vi "Sort sample info metadata.vi"(0 "reference in":refnum<class "metadata.lvclass">, 5 "error in (no error)":errorcluster) -> (14 "reference out":refnum<class "metadata.lvclass">, 16 "Sample info":T1, 19 "error out":errorcluster)   [LabVIEW 2019, in "metadata.lvclass"]
uses:
  metadata.lvclass
  Sample info parameters.ctl
panel:
  out "Array":string[](array[string])
  out "Array 2":i32[](array[numeric])
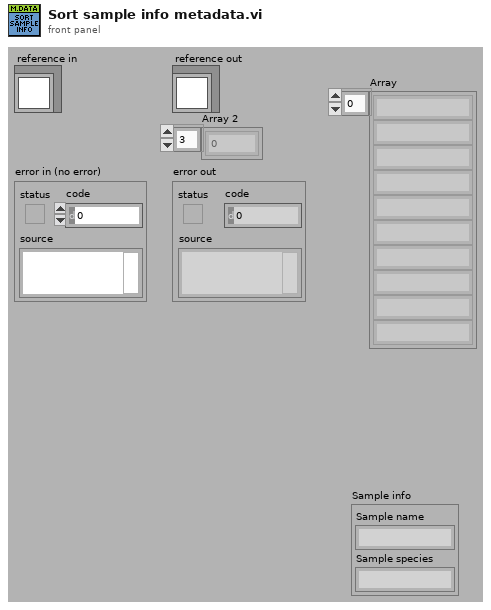
[diagram p1: front panel]
types:
  T1 = typedef "metadata.lvclass/Sample info parameters.ctl" = cluster{"Sample name":string, "Sample species":string}
  T2 = typedef "metadata.lvclass/ObjectAttributesRef.ctl" = refnum<data-value>
  T3 = typedef "metadata.lvclass/ObjectAttributes.ctl" = cluster{"MyAttribute":dbl, "System Control":T4, "file info":T5, "Sample info":T1, "Cantilever info":T6, "XYZ piezos":T7, "Mapping":T8, "Fcurve segment":T9[], "Fast fpga segment":T11, "Chirp":T12, "precision (6)":i16, "width (-)":i16, "Metadata":T13, "config filepath":path, "Section names []":string[], "Property names []":string[], "nb elements":u16}
  T4 = typedef "metadata.lvclass/System control parameters.ctl" = cluster{"FPGA SW version":string, "TDMS file version":string, "Instrument":string, "Instrument model":string, "Instrument scanner":string, "Instrument clockrate (Mhz)":string, "Instrument tick time (us)":string}
  T5 = typedef "metadata.lvclass/File info parameters.ctl" = cluster{"Time Stamp":timestamp, "Filename":string, "Filepath":path, "User":string, "Experiment_name":string, "Curve_id":string, "number_segments":u8, "number_consecutive_scans":u32}
  T6 = typedef "metadata.lvclass/Cantilever info parameters.ctl" = cluster{"spring constant calib method":string, "invOLS calib method":string, "thermal calib deflection channel":string, "model":string, "shape":string, "tip geometry":string, "Laser sum (V)":dbl, "Laser power (mA)":dbl, "invOLS_(nm/V)":dbl, "spring constant nominal (N/m)":dbl, "spring constant calib (N/m)":dbl, "resosnance frequency air calib (Hz)":dbl, "resosnance frequency calib (Hz)":dbl, "quality factor":dbl, "Acoefficident_GCI_(nN.s^1.3/m)":dbl, "half angle (deg)":dbl, "tip radius (m)":dbl, "tip height (m)":dbl, "system mount angle (deg)":dbl}
  T7 = typedef "metadata.lvclass/XYZ piezos parameters.ctl" = cluster{"X stage piezo sensitivity (nm/V)":dbl, "X stage piezo gain":dbl, "X velocity (V/tick)":dbl, "X closed loop":bool, "Y stage piezo sensitivity (nm/V)":dbl, "Y stage piezo gain":dbl, "Y velocity (V/tick)":dbl, "Y closed loop":bool, "Z stage piezo sensitivity (nm/V)":dbl, "Z stage piezo gain":dbl, "Z closed loop":bool, "X position (V)":dbl, "Y position (V)":dbl}
  T8 = typedef "metadata.lvclass/Mapping parameters.ctl" = cluster{"Mapping":bool, "index":u16, "position row":u16, "position column":u16, "next position row":i16, "next position column":i16, "X initial position (V)":dbl, "Y initial position (V)":dbl, "X step size (V)":dbl, "Y step size (V)":dbl}
  T9 = typedef "metadata.lvclass/Fcurve segment.ctl" = cluster{"type":T10, "fast_fpga_trigger":bool, "nb":u8, "duration (ticks)":i64, "nb points":i32, "sampling rate (S/s)":u32, "Zpiezo control out":string, "initial deflection (V)":dbl, "relative setpoint":bool, "setpoint on":bool, "setpoint (V)":dbl, "setpoint trigger channel":string, "velocity (V/tick)":dbl, "Z position setpoint trigger (V)":dbl, "Z retract length (V)":dbl, "dec factor":u32}
  T10 = typedef "metadata.lvclass/Segment type--combobox.ctl" = string
  T11 = typedef "metadata.lvclass/fast fpga segment parameters.ctl" = cluster{"Fast start time trigger":timestamp, "nb_points":u32, "sampling_rate_(S/s)":u32, "duration_(ticks)":u32}
  T12 = typedef "metadata.lvclass/Chirp added parameters.ctl" = cluster{"f start (Hz)":dbl, "f end (Hz)":dbl, "Sweep type":string}
  T13 = typedef "metadata.lvclass/Metadata output --cluster.ctl" = cluster{"Property Names":string[], "Property Values":variant[]}
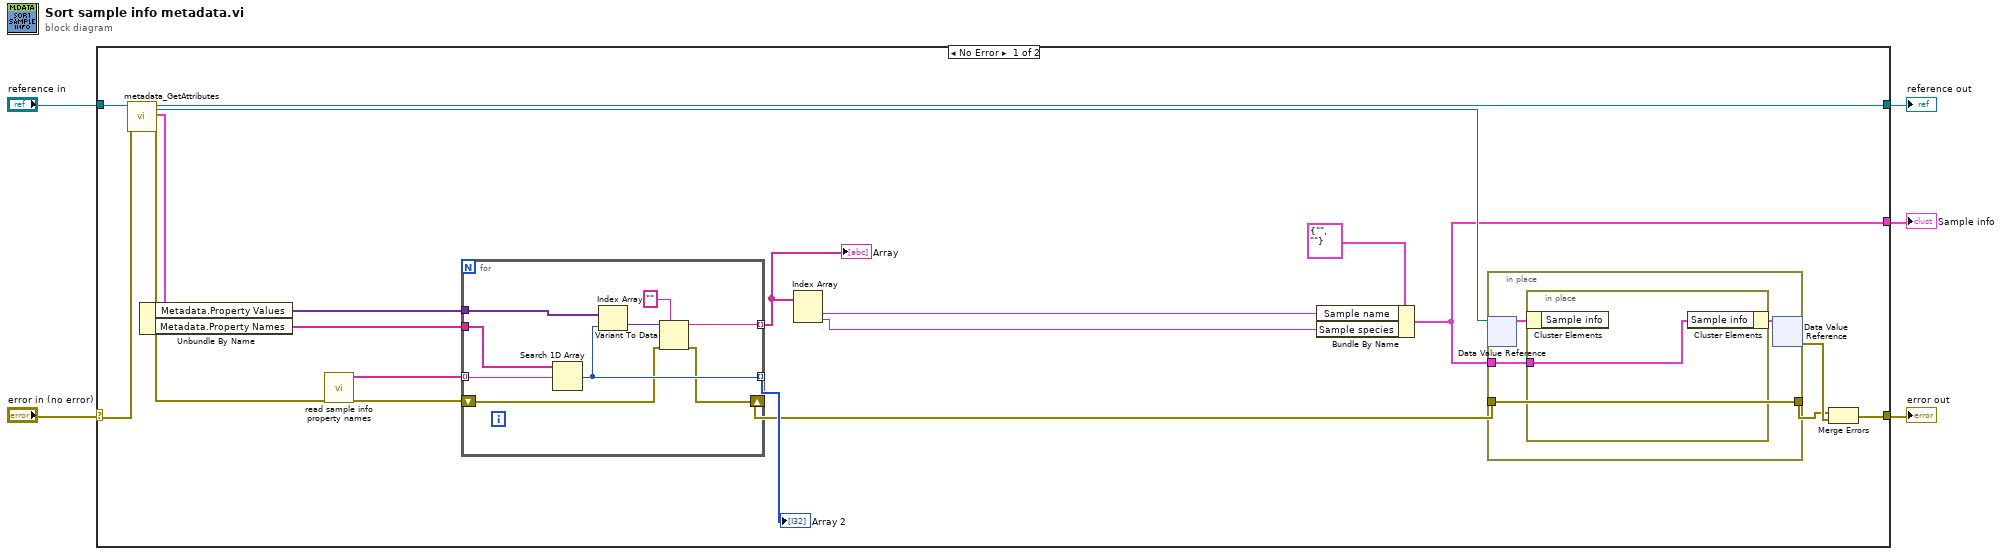
[diagram p0: block diagram]
diagram:
  n1 = case shown="No Error" "error in (no error)" {
    selector: "error in (no error)" -> [w21 w41]
    tunnel: [w25 w41] -> w4
    tunnel: [w20 w40] -> w2
    tunnel: "reference in" -> [w22 w40]
    tunnel: [w12 _] -> w1
    frame No Error {
      n2 = call "metadata_GetAttributes.vi"("reference in"=w22, "error in (no error)"=w21) -> ("reference out"=w20:refnum<class "metadata.lvclass">, "attributes ref"=w19:T2, "attributes"=w18:T3, "error out"=w8:errorcluster)  [unwired: 14 in]
      n3 = Unbundle By Name(w18) -> ("Metadata.Property Values"=w14:variant[], "Metadata.Property Names"=w17:string[])
      n4 = call "read sample info property names.vi"("error in (no error)"=w8) -> ("Sample info"=w6:string[], "error out"=w7:errorcluster)  [unwired: 17 in]
      n5 = for {
        tunnel: w6 -> [w34] mode=indexing
        tunnel: [w31] -> w16 mode=indexing
        shift-right: [w27] -> w15
        shift-left: w7 -> [w28]
        tunnel: w17 -> [w33]
        tunnel: w14 -> [w32]
        tunnel: [w29] -> w13 mode=indexing
        n6 = Search 1D Array(1D array=w33, element=w34) -> (index of element=w31:i32)  [unwired: 1 in]
        n7 = Index Array(array=w32, index=w31) -> (element=w30:variant)
        n8 = Variant To Data(error in=w28, type="", Variant=w30) -> (data=w29:string, error out=w27:errorcluster)
      }
      "Array 2" <- w16
      "Array" <- w13
      n9 = Index Array(array=w13) -> (element #1=w10:string, element #2=w9:string)  [unwired: 2 in]
      n10 = Bundle By Name(cluster=T1 {"Sample name"="", "Sample species"=""} ("Sample info"), "Sample name"=w10, "Sample species"=w9) -> (w12:T1)
      n11 = in-place {
        in-place-border: w15 -> [w36]
        in-place-border: [w36] -> w23
        in-place-border: w12 -> [w35]
        n12 = in-place-dvr #1(w19) -> (w37:T3)  [unwired: 1 out]
        n13 = in-place {
          in-place-border: w35 -> [w39]
          n14 = in-place-cluster #2(w37) -> ()  [unwired: 1 out]
          n15 = in-place-cluster #2("Sample info"=w39) -> (w38:T3)
        }
        n16 = in-place-dvr #1(w38) -> (w24:errorcluster)  [unwired: 1 out]
      }
      n17 = Merge Errors(w23, w24) -> (w25:errorcluster)
    }
    frame Error {
    }
  }
  "error out" <- w4
  "reference out" <- w2
  "Sample info" <- w1
